vi "读取窗口外边框.vi"(8 "错误输入（无错误）":errorcluster, 11 "引用":refnum<vi>) -> (0 "错误输出":errorcluster, 2 "前面板窗口:窗口边界":T1, 3 "引用输出":refnum<vi>)   [LabVIEW 8.6, in "窗口操作.lvlib"]
uses:
  <vilib>/Utility/miscctls.llb/LVRectTypeDef.ctl
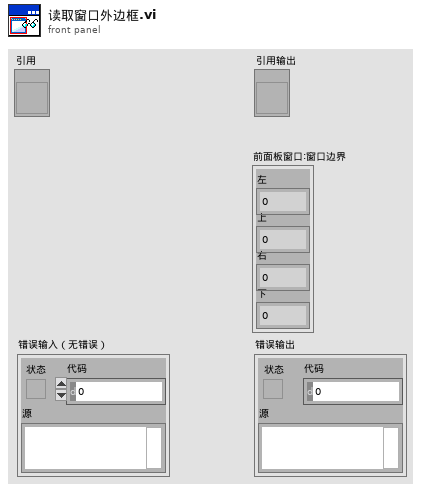
[diagram p1: front panel]
types:
  T1 = typedef "LVRectTypeDef.ctl" = cluster{"Left":i16, "Top":i16, "Right":i16, "Bottom":i16}
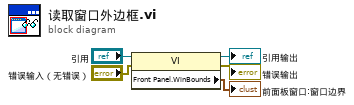
[diagram p0: block diagram]
diagram:
  n1 = property class="VI"(reference="引用", error in="错误输入（无错误）") -> (reference out=→"引用输出":refnum<vi>, error out=→"错误输出":errorcluster, "Front Panel.WinBounds"=→"前面板窗口:窗口边界":T1)
